vi "RFmxSpecAn Global.vi"() -> ()   [LabVIEW 2018]
panel:
  out "Stop?":bool
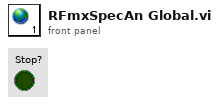
[diagram p1: front panel]
diagram:
